vi "SLSC Add Command Section.vi"(8 "error in (no error)":errorcluster, 9 "Physical Channel":string, 10 "commands":T2[](array[typedef]), 11 "Parent Ref in":T1 format="%.0x") -> (0 "error out":errorcluster, 3 "Parent Ref out":T1 format="%.0x")   [LabVIEW 2015, in "SLSC EDS System Explorer.lvlib"]
uses:
  System Explorer/SLSC EDS System Explorer.lvlib
  SLSC EDS API/JSON parsing/command.ctl
  <vilib>/NI Veristand/Custom Device API/Custom Device Item Ref.ctl
  Shared/Constants.vi
  Shared/SLSC EDS Shared.lvlib
  SLSC CD System Explorer.lvlib
  <vilib>/NI VeriStand/Custom Device API/Custom Device API.lvlib
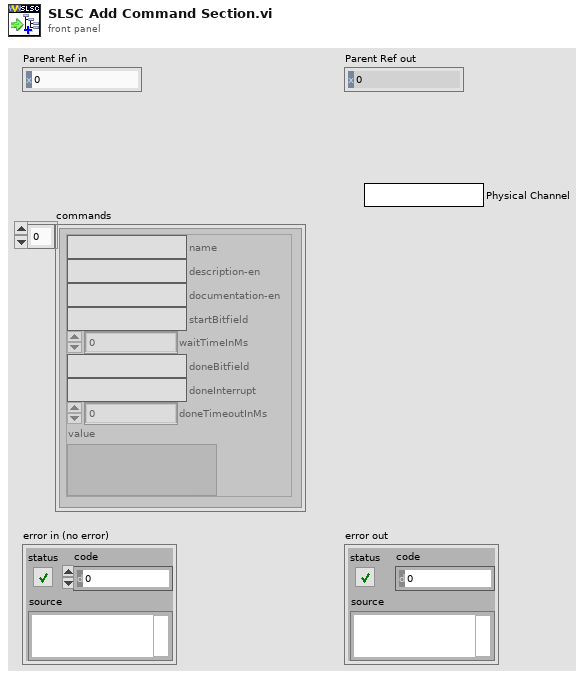
[diagram p1: front panel]
types:
  T1 = typedef "Custom Device API.lvlib/Custom Device Item Ref.ctl" = u64
  T2 = typedef "command.ctl" = cluster{"name":string, "description-en":string, "documentation-en":string, "startBitfield":string, "waitTimeInMs":i32, "doneBitfield":string, "doneInterrupt":string, "doneTimeoutInMs":i32, "value":variant}
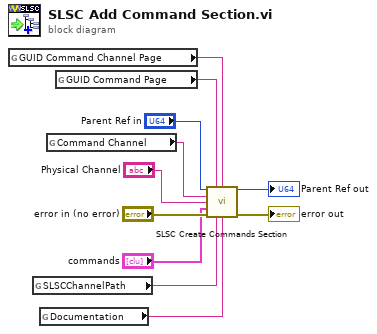
[diagram p0: block diagram]
diagram:
  n1 = global read "Constants.vi" "GUID Command Channel Page"() -> (w3:string)
  n2 = global read "Constants.vi" "SLSCChannelPath"() -> (w7:string)
  n3 = global read "Constants.vi" "Documentation"() -> (w5:string)
  n4 = global read "Constants.vi" "Command Channel"() -> (w1:string)
  n5 = global read "Constants.vi" "GUID Command Page"() -> (w4:string)
  n6 = call "SLSC Create Commands Section.vi"("Parent Ref in"="Parent Ref in", "GUID Command Page"=w4, "GUID Command Channel Page"=w3, "Command Channel"=w1, "Physical Channel"="Physical Channel", "commands"="commands", "error in (no error)"="error in (no error)", "SLSCChannelPath"=w7, "Documentation"=w5) -> ("Parent Ref out"=→"Parent Ref out":T1, "error out"=→"error out":errorcluster)  [unwired: 5 in]
